vi "Add New Test.vi"(7 "Micropulse # In":i32, 8 "error in (no error)":errorcluster, 11 "Test Parameters":T1 {"Rx Channel" min=1 max=1024; "Tx Channel" min=1 max=1024}) -> (0 "error out":errorcluster, 2 "Tx Channel out":u32, 3 "Test No. out":u32, 5 "Micropulse # Out":i32)   [LabVIEW 2026, in "MicroPulse_Driver.lvlib"]
uses:
  MicroPulse_Driver.lvlib
  <instrlib>/MicroPulse/Public/Data/Datatypes/MP - test parameters.ctl
panel:
  out "Rx Channel out":u32
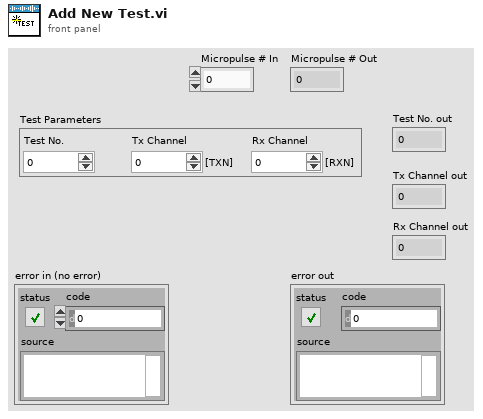
[diagram p1: front panel]
types:
  T1 = typedef "MicroPulse_Driver.lvlib/MP - test parameters.ctl" = cluster{"Test No.":u32, "Tx Channel":u32, "Rx Channel":u32}
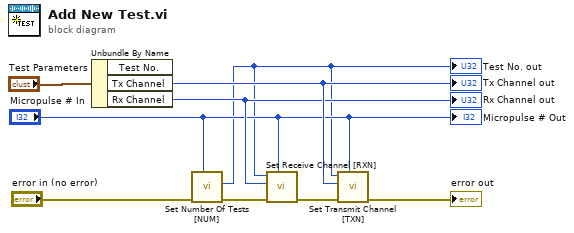
[diagram p0: block diagram]
diagram:
  n1 = Unbundle By Name("Test Parameters") -> ("Tx Channel"=w9:u32, "Rx Channel"=w4:u32)  [unwired: 1 out]
  "Tx Channel out" <- w9
  "Rx Channel out" <- w4
  n2 = call "Set Number Of Tests [NUM].vi"("Micropulse # In"="Micropulse # In", "error in (no error)"="error in (no error)") -> ("error out"=w6:errorcluster, "Test No. Added"=w1:u32)  [unwired: 7 in, 1 out]
  "Test No. out" <- w1
  n3 = call "Set Transmit Channel [TXN].vi"("Micropulse # In"="Micropulse # In", "error in (no error)"=w6, "Channel Number"=w9, "Test Number"=w1) -> ("error out"=w5:errorcluster)  [unwired: 6 in, 1 out]
  n4 = call "Set Receive Channel [RXN].vi"("Micropulse # In"="Micropulse # In", "error in (no error)"=w5, "Channel Number"=w4, "Test Number"=w1) -> ("error out"=→"error out":errorcluster)  [unwired: 6 in, 1 out]
  "Micropulse # Out" <- "Micropulse # In"
